vi "StateNode_GOOPKernel.vi"(0 "Ref in":i32, 1 "Data in":T6, 2 "Data shared in":T2, 3 "VI ref":string, 4 "Dynamic VI path":path, 5 "Subclass folders":path[](array[path]), 6 "Subclass names":string[](array[string]), 7 "error in (no error)":errorcluster, 8 "Action":T5, 9 "Subclass?":bool, 10 "Object name":string, 11 "Dynamic VI name":string, 13 "First try?":bool, 15 "Occurrence":refnum<k4>, 17 "Occurrence shared":refnum<k4>) -> (14 "Occurrence out":refnum<k4>, 16 "# of objects":i32, 18 "Class\nstatistics":T1, 19 "IsSubclass?":bool, 20 "Ref out":i32, 21 "Data out":T6, 22 "Data shared out":T2, 23 "VI ref out":string, 24 "Dynamic VI path out":path, 25 "Exists?":bool, 26 "Data locked?":bool, 27 "error out":errorcluster)   [LabVIEW 2016, in "StateNode.lvclass"]
doc: "This VIs manages objects of the StateNode.\n\n[GOOP 2.0.15]"
uses:
  <resource>/Framework/Providers/Open_GDS/UML/StateNode_class/StateNode.lvclass
  <resource>/Framework/Providers/Open_GDS/UML/RectangularNode_class/RectangularNode.lvclass
  <resource>/Framework/Providers/Open_GDS/UML/AbstractNode_class/AbstractNode.lvclass
  <vilib>/addons/_goop3.llb/3GOOPStates.ctl
  <vilib>/addons/_goop3.llb/3GOOPClassStatistics.ctl
  <resource>/Framework/Providers/Open_GDS/UML/AbstractNode_class/protected/ClassAttributes.ctl
  <resource>/Framework/Providers/Open_GDS/UML/RectangularNode_class/protected/ClassAttributes.ctl
  <resource>/Framework/Providers/Open_GDS/UML/StateNode_class/protected/ClassAttributes.ctl
  <resource>/Framework/Providers/Open_GDS/UML/StateNode_class/protected/ObjectAttributes.ctl
  <resource>/Framework/Providers/Open_GDS/UML/MultiLineString_class/MultiLineString.lvclass
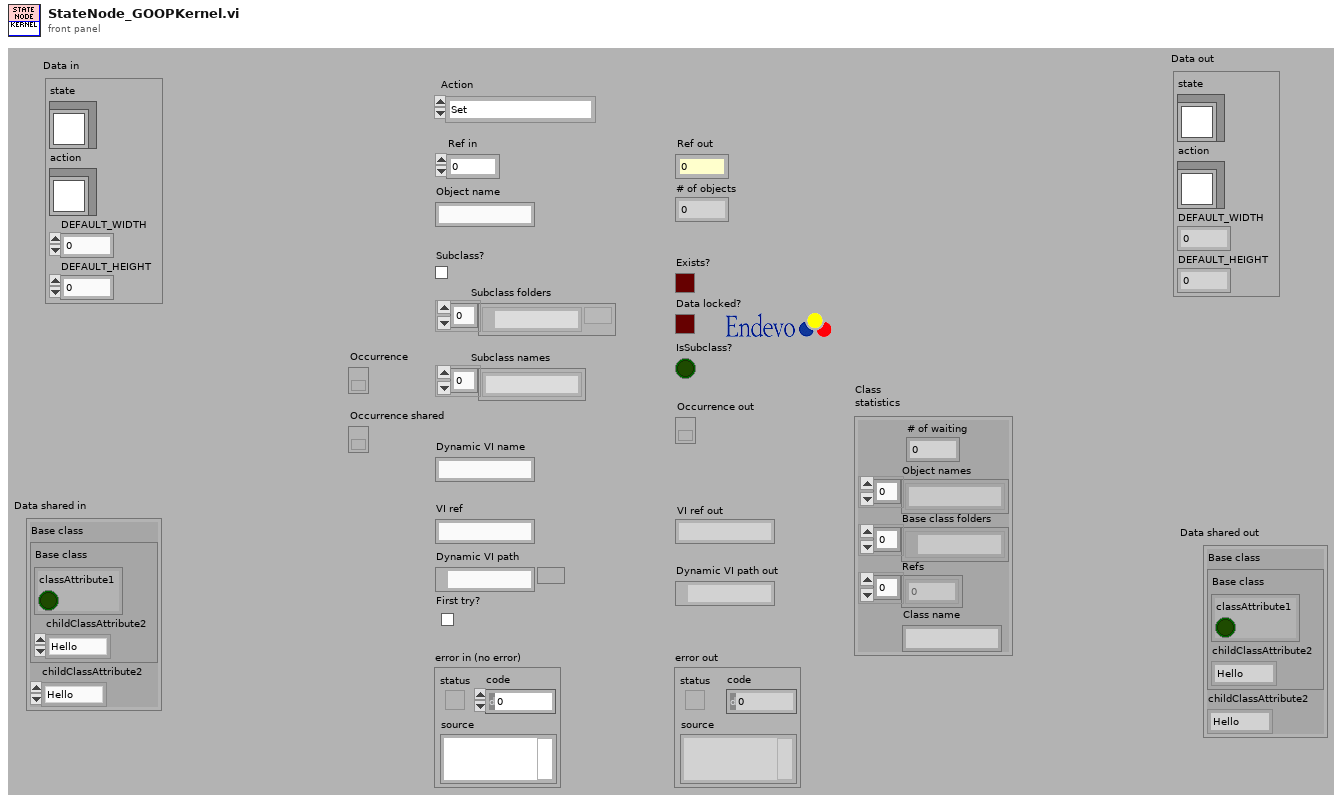
[diagram p1: front panel]
types:
  T1 = typedef "3GOOPClassStatistics.ctl" = cluster{"# of waiting":u32, "Object names":string[], "Base class folders":path[], "Refs":i32[], "Class name":string}
  T2 = typedef "StateNode.lvclass/ClassAttributes.ctl" = cluster{"Base class":T3, "childClassAttribute2":enum16{"Hello", "Goodbye"}}
  T3 = typedef "RectangularNode.lvclass/ClassAttributes.ctl" = cluster{"Base class":T4, "childClassAttribute2":enum16{"Hello", "Goodbye"}}
  T4 = typedef "AbstractNode.lvclass/ClassAttributes.ctl" = cluster{"classAttribute1":bool}
  T5 = typedef "3GOOPStates.ctl" = enum16{"Set", "Get", "New", "Delete", "Clear", "Test and get", "Unlock data", "Information", "Look up existing", "New or look up existing", "Test and get shared", "Get shared", "Set shared", "Unlock shared", "Find dynamic method", "Register dynamic method", "Preload dynamic method", "Probe", "Cast to more generic", "Cast to more specific"}
  T6 = typedef "StateNode.lvclass/ObjectAttributes.ctl" = cluster{"state":refnum<class "MultiLineString.lvclass">, "action":refnum<class "MultiLineString.lvclass">, "DEFAULT_WIDTH":i32, "DEFAULT_HEIGHT":i32}
  T7 = typedef "RectangularNode.lvclass/ObjectAttributes.ctl" = cluster{"Base class":T8, "bounds":T9}
  T8 = typedef "AbstractNode.lvclass/ObjectAttributes.ctl" = cluster{"parent":refnum<class "AbstractNode.lvclass">, "children":refnum<class "AbstractNode.lvclass">[], "Hidden":bool}
  T9 = typedef "Rectangle Rectangle2D.ctl" = cluster{"x":dbl, "y":dbl, "width":dbl, "height":dbl}
  T10 = typedef "RectangularNode.lvclass/ObjectAttributes.ctl" = cluster{"bounds":T9}
  T11 = cluster{"Name":string, "Subclass":bool, "Class":string}[]
  T12 = cluster{"Name":string, "Subclass":bool, "Class":string}
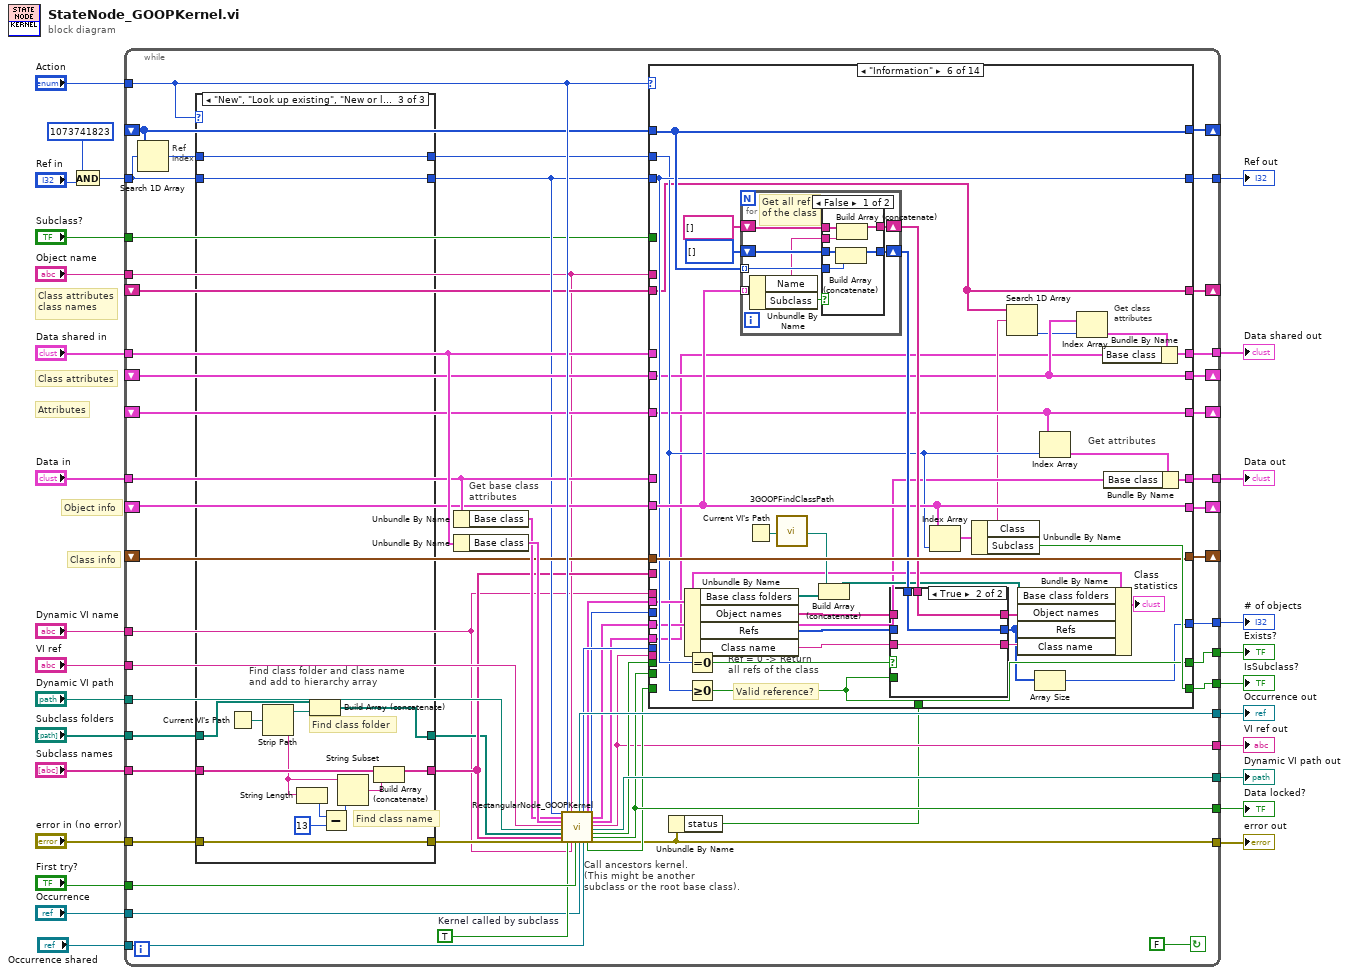
[diagram p0: block diagram]
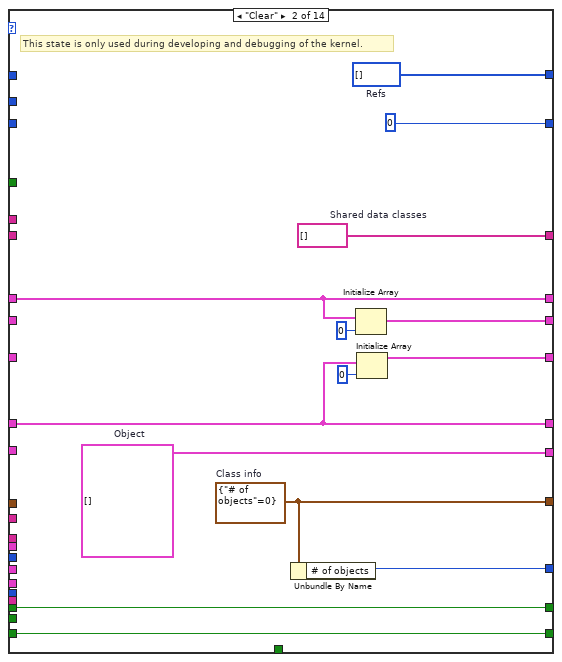
[diagram p3: hidden frame]
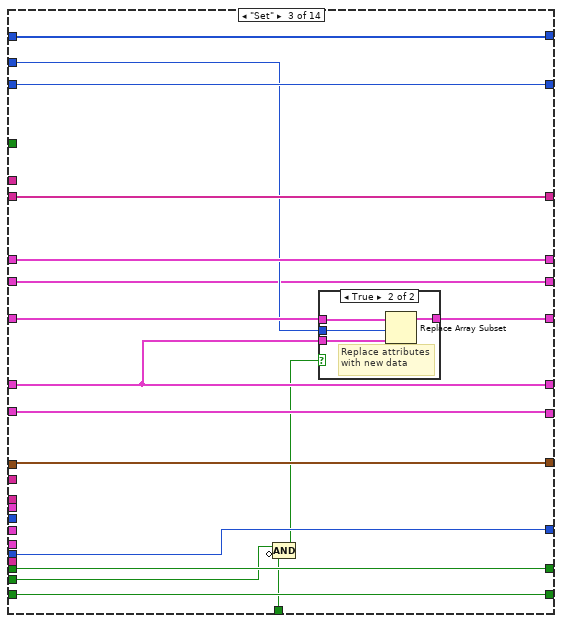
[diagram p4: hidden frame]
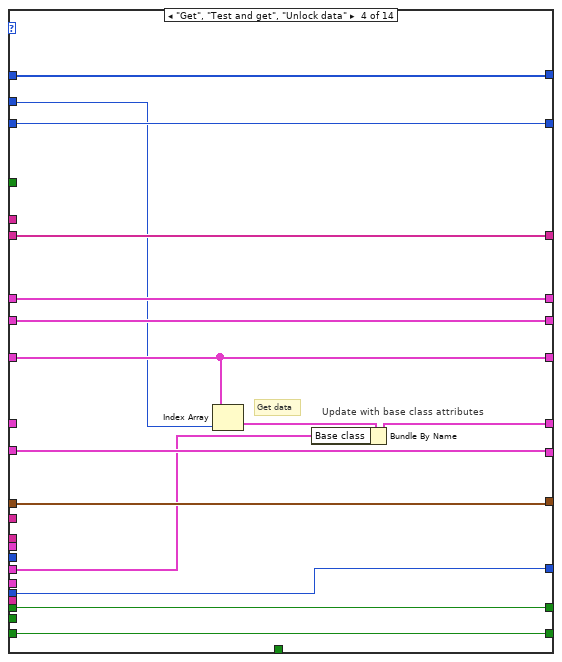
[diagram p6: hidden frame]
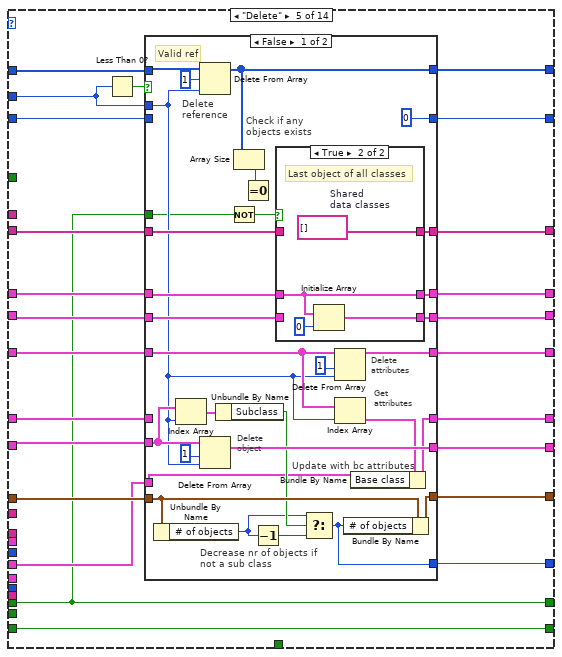
[diagram p7: hidden frame]
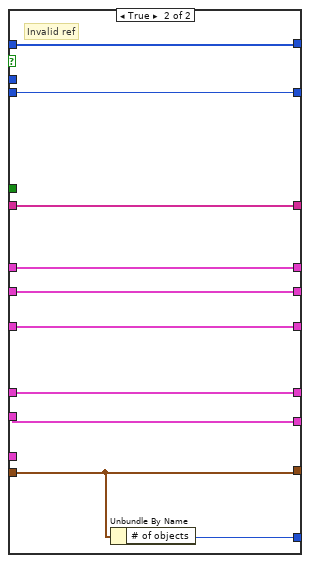
[diagram p9: hidden frame]
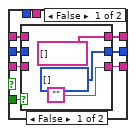
[diagram p10: hidden frame]
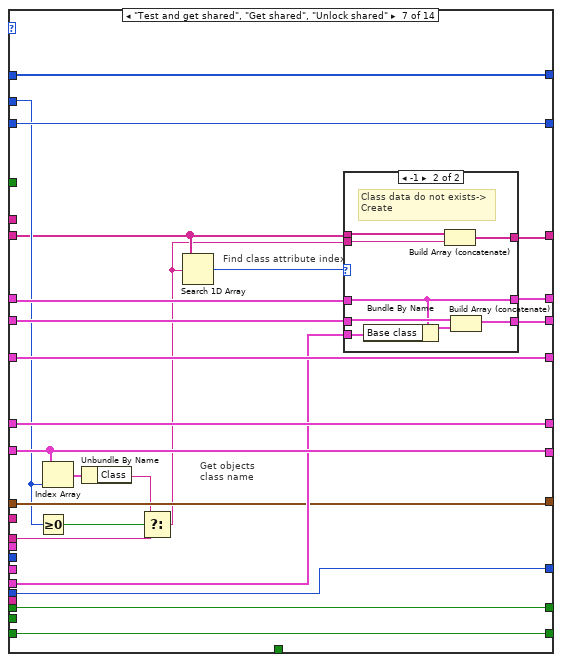
[diagram p13: hidden frame]
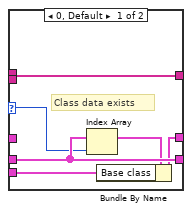
[diagram p14: hidden frame]
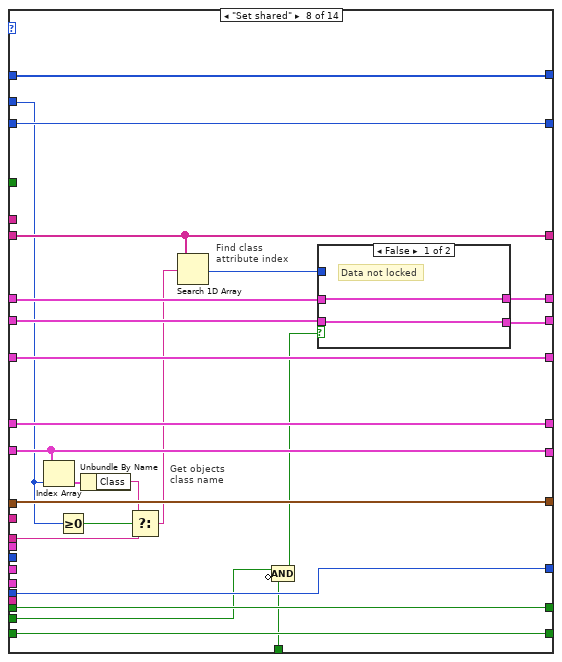
[diagram p15: hidden frame]
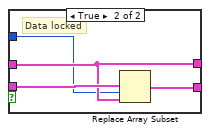
[diagram p16: hidden frame]
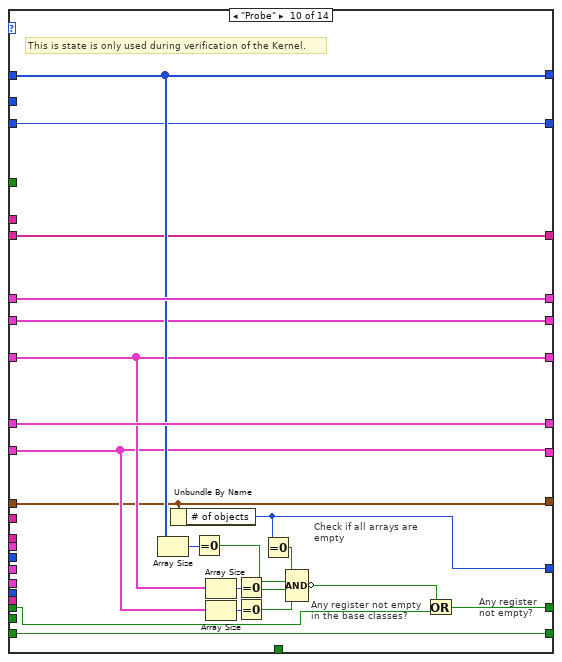
[diagram p18: hidden frame]
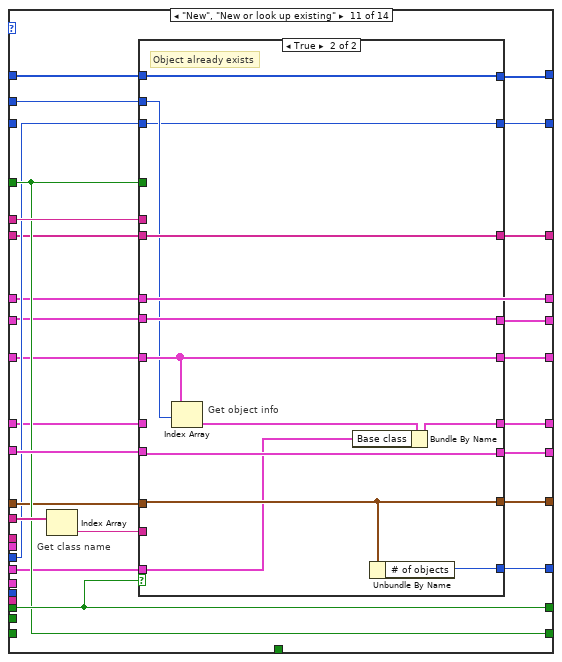
[diagram p19: hidden frame]
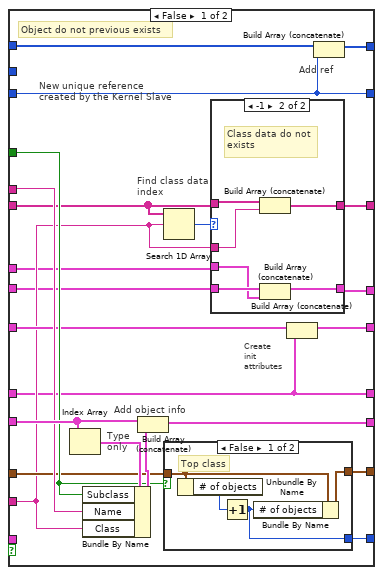
[diagram p20: hidden frame]
diagram:
  # "Class attributes\nclass names"
  # "Attributes"
  # "Class attributes"
  # "Class info"
  # "Object info"
  n1 = And(x=1073741823 ("x .and. y?"), y="Ref in") -> (x .and. y?=w3:i32)
  n2 = while {
    tunnel: [w56] -> w7
    tunnel: [w58] -> w8
    tunnel: "First try?" -> [w79]
    shift-left: _ -> [w44]
    shift-right: [w78] -> _
    tunnel: [w65] -> w10
    tunnel: [w40] -> w11
    tunnel: "Subclass folders" -> [w67]
    tunnel: "Subclass names" -> [w68]
    tunnel: "VI ref" -> [w70]
    tunnel: [w55] -> w15
    tunnel: "Dynamic VI path" -> [w69]
    tunnel: [w33] -> w17
    tunnel: "Dynamic VI name" -> [w34]
    tunnel: "Data shared in" -> [w75]
    shift-left: _ -> [w60]
    shift-right: [w77] -> _
    shift-left: _ -> [w63]
    shift-right: [w64] -> _
    shift-left: _ -> [w62]
    shift-right: [w61] -> _
    tunnel: [w54] -> w6
    tunnel: "Object name" -> [w35]
    tunnel: [w32] -> w21
    tunnel: "error in (no error)" -> [w80]
    shift-left: _ -> [w46]
    shift-right: [w82] -> _
    tunnel: "Subclass?" -> [w36]
    tunnel: [w43] -> w24
    tunnel: [w81] -> w25
    tunnel: w3 -> [w47]
    shift-left: _ -> [w59]
    shift-right: [w76] -> _
    tunnel: [w66] -> w26
    tunnel: "Action" -> [w83]
    tunnel: "Data in" -> [w72]
    tunnel: "Occurrence" -> [w30]
    tunnel: "Occurrence shared" -> [w29]
    stop <- FALSE continue-if-true
    w39 = TRUE  # Kernel called by subclass
    # "Call ancestors kernel.\n(This might be another\nsubclass or the root base class)."
    # "Ref\nindex"
    # "Get base class\nattributes"
    n3 = Search 1D Array(1D array=w46, element=w47) -> (index of element=w48:i32)  [unwired: 1 out]
    n4 = case shown="\"New\", \"Look up existing\", \"New or look up existing\", \"Cast to more generic\", \"Cast to more specific\"" w83 {
      tunnel: w80 -> [w668 w675 w687]
      tunnel: [w667 w675 w687] -> w74
      tunnel: w68 -> [w664 w674 w680]
      tunnel: w67 -> [w665 w673 w679]
      tunnel: [w664 w674 w681] -> w38
      tunnel: [w665 w673 w678] -> w37
      tunnel: w48 -> [w663 w672 w689]
      tunnel: w47 -> [w666 w671 w688]
      tunnel: [w666 w671 w688] -> w45
      tunnel: [w663 w672 w689] -> w42
      frame "Set", "Get", "Delete", "Test and get", "Unlock data", "Find dynamic method", "Register dynamic method" {
        # "Check if reference\nis valid"
        n5 = Less Than 0?(x=w663) -> (x < 0?=w669:bool)
        n6 = call <vilib>:"3GOOPSetError.vi"("ref"=w666, "error"=w669, "error in (no error)"=w668, "call depth"=1) -> ("error out"=w667:errorcluster)  [unwired: 2 in, 13 out]
      }
      frame "Clear", "Information", "Test and get shared".."Unlock shared", "Preload dynamic method", "Probe", Default {
      }
      frame "New", "Look up existing", "New or look up existing", "Cast to more generic", "Cast to more specific" {
        # "Find class folder and class name\nand add to hierarchy array"
        # "Find class folder"
        # "Find class name"
        n7 = Current VI's Path() -> (path=w686:path)
        n8 = Strip Path(path=w686) -> (stripped path=w682:path, name=w676:string)
        n9 = String Length(string=w676) -> (length=w685:i32)
        n10 = Build Array (concatenate)(w679, w682) -> (w678:path[])
        n11 = Subtract(x=w685, y=13) -> (x-y=w683:i32)
        n12 = String Subset(string=w676, length (rest)=w683) -> (substring=w677:string)  [unwired: 1 out]
        n13 = Build Array (concatenate)(w680, w677) -> (w681:string[])
      }
    }
    n14 = Unbundle By Name(w72) -> ("Base class"=w71:T7)
    n15 = Unbundle By Name(w75) -> ("Base class"=w73:T3)
    n16 = call <resource>:"RectangularNode_GOOPKernel.vi"("Ref in"=w45, "Data in"=w71, "Data shared in"=w73, "VI ref"=w70, "Dynamic VI path"=w69, "Subclass folders"=w37, "Subclass names"=w38, "error in (no error)"=w74, "Action"=w83, "Subclass?"=w39, "Object name"=w35, "Dynamic VI name"=w34, "First try?"=w79, "Occurrence"=w30, "Occurrence shared"=w29) -> ("Occurrence out"=w58:refnum<k4>, "# of objects"=w57:i32, "Class\nstatistics"=w53:T1, "IsSubclass?"=w41:bool, "Ref out"=w52:i32, "Data out"=w51:T10, "Data shared out"=w50:T3, "VI ref out"=w33:string, "Dynamic VI path out"=w55:path, "Exists?"=w49:bool, "Data locked?"=w43:bool, "error out"=w32:errorcluster)  [unwired: 1 out]
    n17 = Unbundle By Name(w32) -> ("status"=w31:bool)
    n18 = case shown="\"Information\"" w83 {
      tunnel: [w96 w110 w127 w135 w168 w253 w299 w337 w366 w376 w402 w475 w512 w587] -> w82
      tunnel: [w94 0 ("Ref in") w126 w136 w158 w237 w300 w336 w365 w375 w399 w472 w511 w581] -> w81
      tunnel: [w95 w106 w123 w137 w157 w225 w289 w342 w364 w374 w396 w469 w517 w591] -> w78
      tunnel: w75 -> [w93 w102 w122 w139 w167 _ w306 w346 w363 w377 w392 w465 w518 w592]
      tunnel: [w92 w105 w115 w138 w155 w222 w308 w344 w362 w373 w395 w468 w519 w593] -> w77
      tunnel: w72 -> [w90 w103 w116 _ w151 _ w303 w340 w360 w378 w391 w464 w521 w580]
      tunnel: [w91 w104 w125 w145 w164 w229 w304 w341 w361 w372 w398 w471 w516 w590] -> w76
      tunnel: [w90 w103 w116 w143 w152 w228 w303 w340 w360 w378 w388 w461 w521 w579] -> w66
      tunnel: [w93 w102 w122 w139 w166 w223 w307 w347 w363 w377 w392 w465 w518 w592] -> w65
      tunnel: [w88 w99 w120 w147 w160 w250 w296 w338 w358 w369 w404 w477 w524 w597] -> w64
      tunnel: w63 -> [w88 _ w120 w147 w161 w250 w296 w338 w358 w369 w405 w478 w525 w598]
      tunnel: w62 -> [w89 _ w119 w146 w163 w239 w309 w339 w359 w371 w411 w484 w523 w596]
      tunnel: [w89 w101 w119 w146 w162 w239 w309 w339 w359 w371 w410 w483 w522 w595] -> w61
      tunnel: w60 -> [w92 _ w115 w138 w154 w222 w305 w345 w362 w373 w393 w466 w519 w593]
      tunnel: w59 -> [w91 _ w124 w145 w165 w229 w304 w341 w361 w372 w397 w470 w520 w594]
      tunnel: w57 -> [_ _ w118 w141 _ _ w297 w335 w357 _ _ _ w526 _]
      tunnel: [w87 w98 w118 w141 w159 w233 w297 w335 w357 w368 w403 w476 w526 w577] -> w56
      tunnel: [w86 w100 w117 w140 w148 w235 w302 w334 w356 w382 w407 w480 w507 w583] -> w54
      tunnel: w53 -> [_ _ _ _ _ w231 _ _ _ _ _ _ _ _]
      tunnel: w52 -> [w87 _ _ _ _ _ _ _ _ _ w400 w473 _ _]
      tunnel: w51 -> [_ _ _ w142 w153 w226 _ _ _ _ w390 w463 _ w574]
      tunnel: w50 -> [_ _ _ _ _ w219 w298 _ _ _ _ _ _ _]
      tunnel: w49 -> [w86 w100 w117 w140 w148 _ w302 w334 w356 w380 w407 w480 w507 w583]
      tunnel: w46 -> [w96 _ w127 w135 w170 w253 w299 w337 w366 w376 w401 w474 w513 w588]
      tunnel: w45 -> [w94 _ w126 w136 w169 w237 w300 w336 w365 w375 _ _ w511 w582]
      tunnel: w44 -> [w95 _ w123 w137 w156 w225 w291 w342 w364 w374 w394 w467 w517 w591]
      tunnel: w43 -> [_ _ w112 _ _ _ _ w326 _ _ _ _ _ _]
      tunnel: w42 -> [_ _ w121 w134 w149 w230 w295 w330 _ _ w389 w462 w509 w585]
      tunnel: w41 -> [w85 w97 w114 w133 w150 _ w301 w333 w355 w379 _ _ w527 w599]
      tunnel: [w85 w97 w114 w133 w150 w251 w301 w333 w355 w379 w406 w479 w527 w599] -> w40
      tunnel: w38 -> [_ _ _ _ _ _ _ _ _ _ w412 w485 w514 w576]
      tunnel: w36 -> [_ _ _ _ _ _ _ _ _ _ w406 w479 _ w578]
      tunnel: w35 -> [_ _ _ _ _ _ _ _ _ _ w408 w481 _ _]
      tunnel: w34 -> [_ _ _ _ _ _ w292 w331 _ _ _ _ _ _]
      tunnel: w33 -> [_ _ _ _ _ _ _ _ _ _ _ _ w515 w589]
      tunnel: w31 -> [_ _ w113 _ _ _ _ w327 _ _ _ _ _ _]
      frame Default {
      }
      frame "Clear" {
        w99 = cluster{"# of objects":i32} {"# of objects"=0}  # Class info
        w101 = T11 []  # Object
        w106 = string[] []  # Shared data classes
        w110 = i32[] []  # Refs
        # "This state is only used during developing and debugging of the kernel."
        n19 = Unbundle By Name(w99) -> ("# of objects"=w98:i32)
        n20 = Initialize Array(w102, 0 ("Dimension Size")) -> (w105:T2[])
        n21 = Initialize Array(w103, 0 ("Dimension Size")) -> (w104:T6[])
      }
      frame "Set" {
        n22 = Compound Arithmetic op=AND(w112, invert w113) -> (w111:bool)
        n23 = case shown="True" w111 {
          tunnel: w116 -> [_ w132]
          tunnel: w124 -> [w128 w131]
          tunnel: [w128 w130] -> w125
          tunnel: w121 -> [_ w129]
          frame False {
            # "Data not locked!"
          }
          frame True {
            # "Replace attributes\nwith new data"
            n24 = Replace Array Subset(array=w131, new element=w132, index=w129) -> (w130:T6[])
          }
        }
      }
      frame "Get", "Test and get", "Unlock data" {
        # "Update with base class attributes"
        # "Get data"
        n25 = Index Array(array=w145, index=w134) -> (element=w144:T6)
        n26 = Bundle By Name(cluster=w144, "Base class"=w142) -> (w143:T6)
      }
      frame "Delete" {
        n27 = Less Than 0?(x=w149) -> (x < 0?=w171:bool)
        n28 = case shown="False" w171 {
          tunnel: w170 -> [w200 w216]
          tunnel: w169 -> [_ w215]
          tunnel: [w188 w216] -> w168
          tunnel: w167 -> [w185 w213]
          tunnel: [w186 w213] -> w166
          tunnel: w165 -> [w180 w211]
          tunnel: [w198 w211] -> w164
          tunnel: w163 -> [w195 w210]
          tunnel: [w197 w210] -> w162
          tunnel: w161 -> [w192 w218]
          tunnel: [w193 w218] -> w160
          tunnel: [w190 w217] -> w159
          tunnel: [0 w215] -> w158
          tunnel: [w184 w214] -> w157
          tunnel: w156 -> [w183 w214]
          tunnel: [w182 w212] -> w155
          tunnel: w154 -> [w181 w212]
          tunnel: w153 -> [w177 _]
          tunnel: [w179 w209] -> w152
          tunnel: w151 -> [_ w209]
          tunnel: w149 -> [w176 _]
          tunnel: w148 -> [w172 _]
          frame False {
            # "Update with bc attributes"
            # "Delete\nreference"
            # "Check if any\nobjects exists"
            # "Delete\nattributes"
            # "Get\nattributes"
            # "Delete\nobject"
            # "Decrease nr of objects if\nnot a sub class"
            # "Valid ref"
            n29 = Unbundle By Name(w192) -> ("# of objects"=w174:i32)
            n30 = Index Array(array=w195, index=w176) -> (element=w194:T12)
            n31 = Delete From Array(array=w200, length=1 ("Length"), index=w176) -> (array with subset deleted=w188:i32[])  [unwired: 1 out]
            n32 = Delete From Array(array=w195, length=1 ("Length"), index=w176) -> (array with subset deleted=w197:T11)  [unwired: 1 out]
            n33 = Unbundle By Name(w194) -> ("Subclass"=w191:bool)
            n34 = Not(x=w172) -> (.not. x?=w173:bool)
            n35 = Array Size(array=w188) -> (size(s)=w187:i32)
            n36 = Equal To 0?(x=w187) -> ()  [unwired: 1 out]
            n37 = Decrement(x=w174) -> (x-1=w175:i32)
            n38 = case shown="True" w173 {
              tunnel: [w204 w205] -> w186
              tunnel: w185 -> [w204 w205]
              tunnel: w181 -> [w203 _]
              tunnel: [w203 w206] -> w182
              tunnel: w183 -> [w202 _]
              tunnel: [w202 w208] -> w184
              frame False {
              }
              frame True {
                w208 = string[] []  # Shared data classes
                # "Last object of all classes"
                n39 = Initialize Array(w205, 0 ("Dimension Size")) -> (w206:T2[])
              }
            }
            n40 = Select(t=w174, s=w191, f=w175) -> (s? t:f=w190:i32)
            n41 = Delete From Array(array=w180, length=1 ("Length"), index=w176) -> (array with subset deleted=w198:T6[])  [unwired: 1 out]
            n42 = Index Array(array=w180, index=w176) -> (element=w178:T6)
            n43 = Bundle By Name(cluster=w192, "# of objects"=w190) -> (w193:cluster{"# of objects":i32})
            n44 = Bundle By Name(cluster=w178, "Base class"=w177) -> (w179:T6)
          }
          frame True {
            # "Invalid ref"
            n45 = Unbundle By Name(w218) -> ("# of objects"=w217:i32)
          }
        }
      }
      frame "Information" {
        # "Valid reference?"
        # "Ref = 0 -> Return\nall refs of the class"
        # "Get class\nattributes"
        # "Get attributes"
        n46 = Unbundle By Name(w231) -> ("Base class folders"=w242:path[], "Object names"=w246:string[], "Refs"=w247:i32[], "Class name"=w248:string)
        n47 = Equal To 0?(x=w237) -> (x = 0?=w236:bool)
        n48 = Greater Or Equal To 0?(x=w230) -> (x >= 0?=w235:bool)
        n49 = for {
          shift-right: [w278] -> w243
          shift-left: i32[] [] -> [w279]
          tunnel: w253 -> [w277] mode=indexing
          tunnel: w239 -> [w276] mode=indexing
          shift-right: [w273] -> w244
          shift-left: string[] [] ("Object names") -> [w274]
          # "Get all ref\nof the class"
          n50 = Unbundle By Name(w276) -> ("Name"=w272:string, "Subclass"=w275:bool)
          n51 = case shown="False" w275 {
            tunnel: w279 -> [w285 w287]
            tunnel: [w284 w287] -> w278
            tunnel: w277 -> [w283 _]
            tunnel: w274 -> [w282 w286]
            tunnel: [w281 w286] -> w273
            tunnel: w272 -> [w280 _]
            frame False {
              n52 = Build Array (concatenate)(w285, w283) -> (w284:i32[])
              n53 = Build Array (concatenate)(w282, w280) -> (w281:string[])
            }
            frame True {
            }
          }
        }
        n54 = Current VI's Path() -> (path=w240:path)
        n55 = call <vilib>:"3GOOPFindClassPath.vi"("current VI path"=w240) -> ("Class folder"=w238:path)  [unwired: 18 out]
        n56 = Build Array (concatenate)(w238, w242) -> (w241:path[])
        n57 = case shown="True" w236 {
          tunnel: w235 -> [w262 _]
          tunnel: w247 -> [w261 _]
          tunnel: [w260 w270] -> w234
          tunnel: w248 -> [w259 w269]
          tunnel: [w258 w269] -> w249
          tunnel: w246 -> [w257 _]
          tunnel: [w256 w271] -> w245
          tunnel: w244 -> [_ w271]
          tunnel: w243 -> [_ w270]
          frame False {
            n58 = case shown="False" w262 {
              tunnel: w261 -> [_ w268]
              tunnel: [i32[] [] ("Array Constant") w268] -> w260
              tunnel: w259 -> [_ w267]
              tunnel: ["" w267] -> w258
              tunnel: w257 -> [_ w266]
              tunnel: [string[] [] ("Array Constant") w266] -> w256
              frame False {
              }
              frame True {
              }
            }
          }
          frame True {
          }
        }
        n59 = Index Array(array=w239, index=w230) -> (element=w252:T12)
        n60 = Unbundle By Name(w252) -> ("Class"=w224:string, "Subclass"=w251:bool)
        n61 = Search 1D Array(1D array=w225, element=w224) -> (index of element=w221:i32)  [unwired: 1 out]
        n62 = Bundle By Name(cluster=w231, "Base class folders"=w241, "Object names"=w245, "Refs"=w234, "Class name"=w249) -> (→"Class\nstatistics":T1)
        n63 = Array Size(array=w234) -> (size(s)=w233:i32)
        n64 = Index Array(array=w229, index=w230) -> (element=w227:T6)
        n65 = Index Array(array=w222, index=w221) -> (element=w220:T2)
        n66 = Bundle By Name(cluster=w220, "Base class"=w219) -> (w223:T2)
        n67 = Bundle By Name(cluster=w227, "Base class"=w226) -> (w228:T6)
      }
      frame "Test and get shared", "Get shared", "Unlock shared" {
        # "Find class attribute index"
        # "Get objects\nclass name"
        n68 = Greater Or Equal To 0?(x=w295) -> (x >= 0?=w293:bool)
        n69 = Index Array(array=w309, index=w295) -> (element=w310:T12)
        n70 = Unbundle By Name(w310) -> ("Class"=w294:string)
        n71 = Select(t=w294, s=w293, f=w292) -> (s? t:f=w288:string)
        n72 = Search 1D Array(1D array=w291, element=w288) -> (index of element=w290:i32)  [unwired: 1 out]
        n73 = case shown="-1" w290 {
          selector: w290 -> [w311 _]
          tunnel: w305 -> [w316 w324]
          tunnel: [w315 w322] -> w307
          tunnel: [w316 w323] -> w308
          tunnel: w306 -> [_ w322]
          tunnel: w298 -> [w313 w320]
          tunnel: w291 -> [w312 w319]
          tunnel: [w312 w318] -> w289
          tunnel: w288 -> [_ w317]
          frame 0, Default {
            # "Class data exists"
            n74 = Index Array(array=w316, index=w311) -> (element=w314:T2)
            n75 = Bundle By Name(cluster=w314, "Base class"=w313) -> (w315:T2)
          }
          frame -1 {
            # "Class data do not exists->\nCreate"
            n76 = Bundle By Name(cluster=w322, "Base class"=w320) -> (w321:T2)
            n77 = Build Array (concatenate)(w319, w317) -> (w318:string[])
            n78 = Build Array (concatenate)(w324, w321) -> (w323:T2[])
          }
        }
      }
      frame "Set shared" {
        # "Get objects\nclass name"
        # "Find class\nattribute index"
        n79 = Index Array(array=w339, index=w330) -> (element=w348:T12)
        n80 = Greater Or Equal To 0?(x=w330) -> (x >= 0?=w332:bool)
        n81 = Unbundle By Name(w348) -> ("Class"=w329:string)
        n82 = Select(t=w329, s=w332, f=w331) -> (s? t:f=w328:string)
        n83 = Search 1D Array(1D array=w342, element=w328) -> (index of element=w343:i32)  [unwired: 1 out]
        n84 = Compound Arithmetic op=AND(w326, invert w327) -> (w325:bool)
        n85 = case shown="False" w325 {
          tunnel: w346 -> [w350 w352]
          tunnel: w345 -> [w349 w354]
          tunnel: [w349 w353] -> w344
          tunnel: [w350 w352] -> w347
          tunnel: w343 -> [_ w351]
          frame False {
            # "Data not locked"
          }
          frame True {
            # "Data locked"
            n86 = Replace Array Subset(array=w354, new element=w352, index=w351) -> (w353:T2[])
          }
        }
      }
      frame "Find dynamic method".."Preload dynamic method" {
      }
      frame "Probe" {
        # "This is state is only used during verification of the Kernel."
        # "Any register not empty \nin the base classes?"
        # "Any register\nnot empty?"
        # "Check if all arrays are\nempty"
        n87 = Array Size(array=w376) -> (size(s)=w385:i32)
        n88 = Unbundle By Name(w369) -> ("# of objects"=w368:i32)
        n89 = Equal To 0?(x=w385) -> (x = 0?=w370:bool)
        n90 = Array Size(array=w372) -> (size(s)=w387:i32)
        n91 = Array Size(array=w371) -> (size(s)=w386:i32)
        n92 = Equal To 0?(x=w387) -> (x = 0?=w384:bool)
        n93 = Equal To 0?(x=w386) -> (x = 0?=w383:bool)
        n94 = Equal To 0?(x=w368) -> (x = 0?=w367:bool)
        n95 = Compound Arithmetic op=AND(w367, w370, w384, w383) -> (invert w381:bool)
        n96 = Or(x=w381, y=w380) -> (x .or. y?=w382:bool)
      }
      frame "New", "New or look up existing" {
        # "Get class name"
        n97 = Index Array(array=w412) -> (element=w409:string)  [unwired: 1 in]
        n98 = case shown="True" w407 {
          tunnel: w411 -> [w432 w457]
          tunnel: [w431 w457] -> w410
          tunnel: w409 -> [w417 _]
          tunnel: w406 -> [w429 _]
          tunnel: w408 -> [w430 _]
          tunnel: w405 -> [w428 w456]
          tunnel: [w427 w456] -> w404
          tunnel: [w426 w455] -> w403
          tunnel: [w425 w460] -> w402
          tunnel: w401 -> [w424 w460]
          tunnel: w400 -> [w423 w452]
          tunnel: [w423 w452] -> w399
          tunnel: [w422 w454] -> w398
          tunnel: w397 -> [w421 w454]
          tunnel: w391 -> [w414 _]
          tunnel: [w419 w459] -> w396
          tunnel: [w418 w458] -> w395
          tunnel: w394 -> [w413 w459]
          tunnel: w393 -> [w416 w458]
          tunnel: w392 -> [w415 _]
          tunnel: w390 -> [_ w449]
          tunnel: w389 -> [_ w453]
          tunnel: [w414 w450] -> w388
          frame False {
            # "Add ref"
            # "Create\ninit\nattributes"
            # "Add object info"
            # "New unique reference\ncreated by the Kernel Slave"
            # "Find class data\nindex"
            # "Object do not previous exists"
            # "Type\nonly"
            n99 = Index Array(array=w432) -> (element=w434:T12)  [unwired: 1 in]
            n100 = Bundle By Name(cluster=w434, "Subclass"=w429, "Name"=w430, "Class"=w417) -> (w433:T12)
            n101 = Build Array (concatenate)(w432, w433) -> (w431:T11)
            n102 = Search 1D Array(1D array=w413, element=w417) -> (index of element=w420:i32)  [unwired: 1 out]
            n103 = case shown="False" w429 {
              tunnel: w428 -> [w446 w448]
              tunnel: [w445 w448] -> w427
              tunnel: [w443 w447] -> w426
              frame False {
                # "Top class"
                n104 = Unbundle By Name(w446) -> ("# of objects"=w444:i32)
                n105 = Increment(x=w444) -> (x+1=w443:i32)
                n106 = Bundle By Name(cluster=w446, "# of objects"=w443) -> (w445:cluster{"# of objects":i32})
              }
              frame True {
                # "Sub class"
                n107 = Unbundle By Name(w448) -> ("# of objects"=w447:i32)
              }
            }
            n108 = case shown="-1" w420 {
              tunnel: w413 -> [w436 w442]
              tunnel: [w436 w441] -> w419
              tunnel: w417 -> [_ w440]
              tunnel: w416 -> [w435 w439]
              tunnel: [w435 w438] -> w418
              tunnel: w415 -> [_ w437]
              frame 0, Default {
                # "Class data already\nexists"
              }
              frame -1 {
                # "Class data do not\nexists"
                n109 = Build Array (concatenate)(w442, w440) -> (w441:string[])
                n110 = Build Array (concatenate)(w439, w437) -> (w438:T2[])
              }
            }
            n111 = Build Array (concatenate)(w421, w414) -> (w422:T6[])
            n112 = Build Array (concatenate)(w424, w423) -> (w425:i32[])
          }
          frame True {
            # "Get object info"
            # "Object already exists"
            n113 = Index Array(array=w454, index=w453) -> (element=w451:T6)
            n114 = Bundle By Name(cluster=w451, "Base class"=w449) -> (w450:T6)
            n115 = Unbundle By Name(w456) -> ("# of objects"=w455:i32)
          }
        }
      }
      frame "Look up existing" {
        # "Get class name"
        n116 = Index Array(array=w485) -> (element=w482:string)  [unwired: 1 in]
        n117 = case shown="True" w480 {
          tunnel: w484 -> [w487 w503]
          tunnel: [w487 w503] -> w483
          tunnel: w482 -> [_ _]
          tunnel: w479 -> [_ _]
          tunnel: w481 -> [_ _]
          tunnel: w478 -> [w486 w502]
          tunnel: [w486 w502] -> w477
          tunnel: [w494 w501] -> w476
          tunnel: [w493 w506] -> w475
          tunnel: w474 -> [w493 w506]
          tunnel: w473 -> [w492 w498]
          tunnel: [w492 w498] -> w472
          tunnel: [w489 w500] -> w471
          tunnel: w470 -> [w489 w500]
          tunnel: w464 -> [w488 _]
          tunnel: [w491 w505] -> w469
          tunnel: [w490 w504] -> w468
          tunnel: w467 -> [w491 w505]
          tunnel: w466 -> [w490 w504]
          tunnel: w465 -> [_ _]
          tunnel: w463 -> [_ w495]
          tunnel: w462 -> [_ w499]
          tunnel: [w488 w496] -> w461
          frame False {
            # "Object do not previous exists"
            n118 = Unbundle By Name(w486) -> ("# of objects"=w494:i32)
          }
          frame True {
            # "Update with base class attributes"
            # "Get object info"
            # "Object already exists"
            n119 = Index Array(array=w500, index=w499) -> (element=w497:T6)
            n120 = Bundle By Name(cluster=w497, "Base class"=w495) -> (w496:T6)
            n121 = Unbundle By Name(w502) -> ("# of objects"=w501:i32)
          }
        }
      }
      frame "Cast to more generic" {
        n122 = Greater Or Equal To 0?(x=w509) -> (x >= 0?=w508:bool)
        n123 = Compound Arithmetic op=AND(w508, w507) -> (w510:bool)
        n124 = case shown="False" w510 {
          tunnel: w525 -> [w528 w540]
          tunnel: [w528 w539] -> w524
          tunnel: w523 -> [w529 w543]
          tunnel: [w529 w544] -> w522
          tunnel: w520 -> [w530 w545]
          tunnel: [w530 w546] -> w516
          tunnel: w509 -> [_ w542]
          tunnel: w515 -> [_ w538]
          tunnel: w514 -> [_ w537]
          tunnel: w513 -> [w531 w533]
          tunnel: [w531 w532] -> w512
          frame False {
            # "Object not found or error occured in kernel"
          }
          frame True {
            # "Object exists"
            # "New class name"
            n125 = Reverse 1D Array(array=w537) -> (reversed array=w536:string[])
            n126 = Index Array(array=w543, index=w542) -> (element=w534:T12)
            n127 = Index Array(array=w536) -> (element=w535:string)  [unwired: 1 in]
            n128 = Unbundle By Name(w534) -> ("Subclass"=w541:bool)
            n129 = case shown="False" w541 {
              tunnel: [w558 w567] -> w546
              tunnel: w545 -> [w557 w567]
              tunnel: [w556 w572] -> w544
              tunnel: w543 -> [w555 w571]
              tunnel: w542 -> [w547 w568]
              tunnel: w540 -> [w554 w565]
              tunnel: [w553 w564] -> w539
              tunnel: w538 -> [_ w566]
              tunnel: w535 -> [_ w573]
              tunnel: w534 -> [_ w570]
              tunnel: w533 -> [w550 w559]
              tunnel: [w549 w559] -> w532
              frame False {
                w548 = 1 ("Length")
                # "Leaf class -> remove"
                n130 = Unbundle By Name(w554) -> ("# of objects"=w551:i32)
                n131 = Decrement(x=w551) -> (x-1=w552:i32)
                n132 = Bundle By Name(cluster=w554, "# of objects"=w552) -> (w553:cluster{"# of objects":i32})
                n133 = Delete From Array(array=w550, length=w548, index=w547) -> (array with subset deleted=w549:i32[])  [unwired: 1 out]
                n134 = Delete From Array(array=w557, length=w548, index=w547) -> (array with subset deleted=w558:T6[])  [unwired: 1 out]
                n135 = Delete From Array(array=w555, length=w548, index=w547) -> (array with subset deleted=w556:T11)  [unwired: 1 out]
              }
              frame True {
                # "Update object\ninfomation"
                # "Object still exists at this level"
                n136 = Not Equal?(x=w573, y=w566) -> (x != y?=w560:bool)
                n137 = Unbundle By Name(w565) -> ("# of objects"=w562:i32)
                n138 = Increment(x=w562) -> (x+1=w563:i32)
                n139 = Bundle By Name(cluster=w570, "Subclass"=w560, "Class"=w566) -> (w569:T12)
                n140 = Select(t=w562, s=w560, f=w563) -> (s? t:f=w561:i32)
                n141 = Bundle By Name(cluster=w565, "# of objects"=w561) -> (w564:cluster{"# of objects":i32})
                n142 = Replace Array Subset(array=w571, new element=w569, index=w568) -> (w572:T11)
              }
            }
          }
        }
      }
      frame "Cast to more specific" {
        n143 = Greater Or Equal To 0?(x=w585) -> (x >= 0?=w584:bool)
        n144 = Index Array(array=w576) -> (element=w575:string)  [unwired: 1 in]
        n145 = Compound Arithmetic op=AND(w584, w583) -> (w586:bool)
        n146 = case shown="False" w586 {
          tunnel: w598 -> [w612 w649]
          tunnel: [w611 w650] -> w597
          tunnel: w596 -> [w609 w658]
          tunnel: [w610 w661] -> w595
          tunnel: w594 -> [w608 w662]
          tunnel: [w607 w662] -> w590
          tunnel: w585 -> [_ w657]
          tunnel: w589 -> [w601 _]
          tunnel: w588 -> [w616 w660]
          tunnel: [w615 w660] -> w587
          tunnel: w583 -> [w617 _]
          tunnel: w582 -> [w614 w655]
          tunnel: [w613 w655] -> w581
          tunnel: w580 -> [w606 w656]
          tunnel: [w605 w656] -> w579
          tunnel: w578 -> [w604 w645]
          tunnel: [w603 w648] -> w577
          tunnel: w575 -> [w602 w654]
          tunnel: w574 -> [w600 _]
          frame False {
            # "Object not found or error occured in kernel"
            n147 = case shown="True" w617 {
              tunnel: w616 -> [w624 w643]
              tunnel: [w624 w644] -> w615
              tunnel: w614 -> [w623 w642]
              tunnel: [w623 w642] -> w613
              tunnel: w612 -> [w621 w629]
              tunnel: [w621 w630] -> w611
              tunnel: w609 -> [w620 w637]
              tunnel: [w620 w636] -> w610
              tunnel: w608 -> [w618 w641]
              tunnel: [w618 w640] -> w607
              tunnel: w606 -> [w619 w632]
              tunnel: [w619 w633] -> w605
              tunnel: w604 -> [_ w628]
              tunnel: [w622 w625] -> w603
              tunnel: w602 -> [_ w635]
              tunnel: w601 -> [_ w634]
              tunnel: w600 -> [_ w631]
              frame False {
                # "Error"
                n148 = Unbundle By Name(w621) -> ("# of objects"=w622:i32)
              }
              frame True {
                # "Add object info"
                # "Type\nonly"
                # "Add object"
                n149 = Bundle By Name(cluster=w632, "Base class"=w631) -> (w633:T6)
                n150 = Index Array(array=w637) -> (element=w639:T12)  [unwired: 1 in]
                n151 = Bundle By Name(cluster=w639, "Subclass"=w628, "Name"=w634, "Class"=w635) -> (w638:T12)
                n152 = Build Array (concatenate)(w637, w638) -> (w636:T11)
                n153 = Unbundle By Name(w629) -> ("# of objects"=w627:i32)
                n154 = Increment(x=w627) -> (x+1=w626:i32)
                n155 = Select(t=w627, s=w628, f=w626) -> (s? t:f=w625:i32)
                n156 = Bundle By Name(cluster=w629, "# of objects"=w625) -> (w630:cluster{"# of objects":i32})
                n157 = Build Array (concatenate)(w641, w633) -> (w640:T6[])
                n158 = Build Array (concatenate)(w643, w642) -> (w644:i32[])
              }
            }
          }
          frame True {
            # "If object belonged to this class before -> decrease nr of objects"
            # "Update object\ninfomation"
            # "Object exists"
            # "New class name"
            n159 = Index Array(array=w658, index=w657) -> (element=w646:T12)
            n160 = Unbundle By Name(w646) -> ("Subclass"=w653:bool)
            n161 = Compound Arithmetic op=AND(w645, invert w653) -> (w651:bool)
            n162 = Unbundle By Name(w649) -> ("# of objects"=w647:i32)
            n163 = Bundle By Name(cluster=w646, "Subclass"=w645, "Class"=w654) -> (w659:T12)
            n164 = Decrement(x=w647) -> (x-1=w652:i32)
            n165 = Select(t=w652, s=w651, f=w647) -> (s? t:f=w648:i32)
            n166 = Bundle By Name(cluster=w649, "# of objects"=w648) -> (w650:cluster{"# of objects":i32})
            n167 = Replace Array Subset(array=w658, new element=w659, index=w657) -> (w661:T11)
          }
        }
      }
    }
  }
  "Data out" <- w26
  "Ref out" <- w25
  "Data locked?" <- w24
  "error out" <- w21
  "Exists?" <- w6
  "Data shared out" <- w10
  "VI ref out" <- w17
  "Dynamic VI path out" <- w15
  "IsSubclass?" <- w11
  "Occurrence out" <- w8
  "# of objects" <- w7
